vi "initSharedVariables.vi"   [LabVIEW 2017]
uses:
  globalUtilities.vi
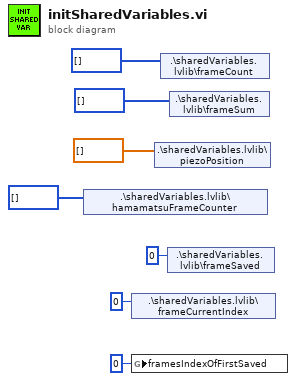
[diagram p0: block diagram]
diagram:
  n1 = shared-variable ".\\sharedVariables.lvlib\\hamamatsuFrameCounter"(u32[] []) -> ()  [unwired: 1 in, 1 out]
  n2 = shared-variable ".\\sharedVariables.lvlib\\frameCurrentIndex"(0 ("frameCurrentIndex")) -> ()  [unwired: 1 in, 1 out]
  n3 = global write "globalUtilities.vi" "framesIndexOfFirstSaved"(0 ("framesIndexOfFirstSaved")) -> ()
  n4 = shared-variable ".\\sharedVariables.lvlib\\piezoPosition"(dbl[] []) -> ()  [unwired: 1 in, 1 out]
  n5 = shared-variable ".\\sharedVariables.lvlib\\frameCount"(i32[] []) -> ()  [unwired: 1 in, 1 out]
  n6 = shared-variable ".\\sharedVariables.lvlib\\frameSaved"(u32 0 ("frameSaved")) -> ()  [unwired: 1 in, 1 out]
  n7 = shared-variable ".\\sharedVariables.lvlib\\frameSum"(i64[] []) -> ()  [unwired: 1 in, 1 out]
